vi "ReadVirtualSetup.vi"(8 "error in (no error)":errorcluster, 11 "Project.lvclass In":refnum<class "Project.lvclass">) -> (0 "error out":errorcluster, 2 "VirtualTypeData":T1={"Search Name"="", "Start X"=0.0, "Increase X"=0.0, "X Step"=1, "Start Y"=0.0, "Increase Y"=0.0, "Y Step"=1, "Sensor"=0} {"Y Step" min=1 step=1; "X Step" min=1 step=1}, 3 "Project.lvclass Out":refnum<class "Project.lvclass">)   [LabVIEW 2014, in "Project.lvclass"]
uses:
  Project.lvclass
  Virtual/Control/AllVirtualTypeData.ctl
  VirtualSetupDataTypeDefine.ctl
  Project.lvclass/Project.ctl
  Virtual/VirtualOrigin.lvclass
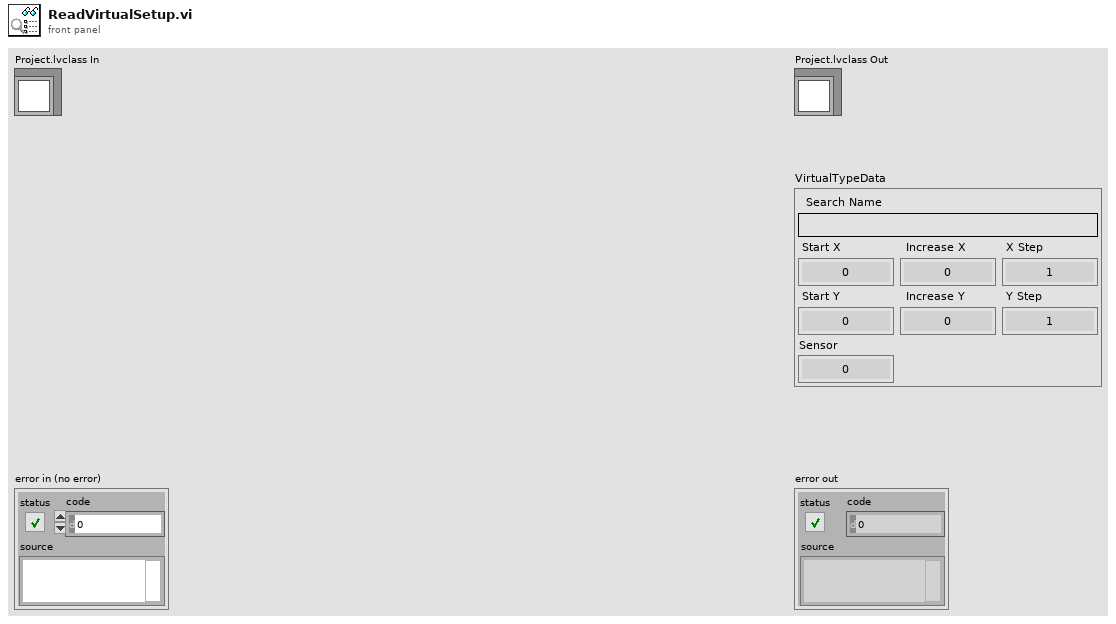
[diagram p1: front panel]
types:
  T1 = typedef "VirtualOrigin.lvclass/AllVirtualTypeData.ctl" = cluster{"Search Name":string, "Start X":dbl, "Increase X":dbl, "X Step":i32, "Start Y":dbl, "Increase Y":dbl, "Y Step":i32, "Sensor":i32}
  T2 = typedef "Project.lvclass/VirtualSetupDataTypeDefine.ctl" = T1[]
  T3 = typedef "Project.lvclass/ProjectDataTableTypeDefine.ctl" = string[][]
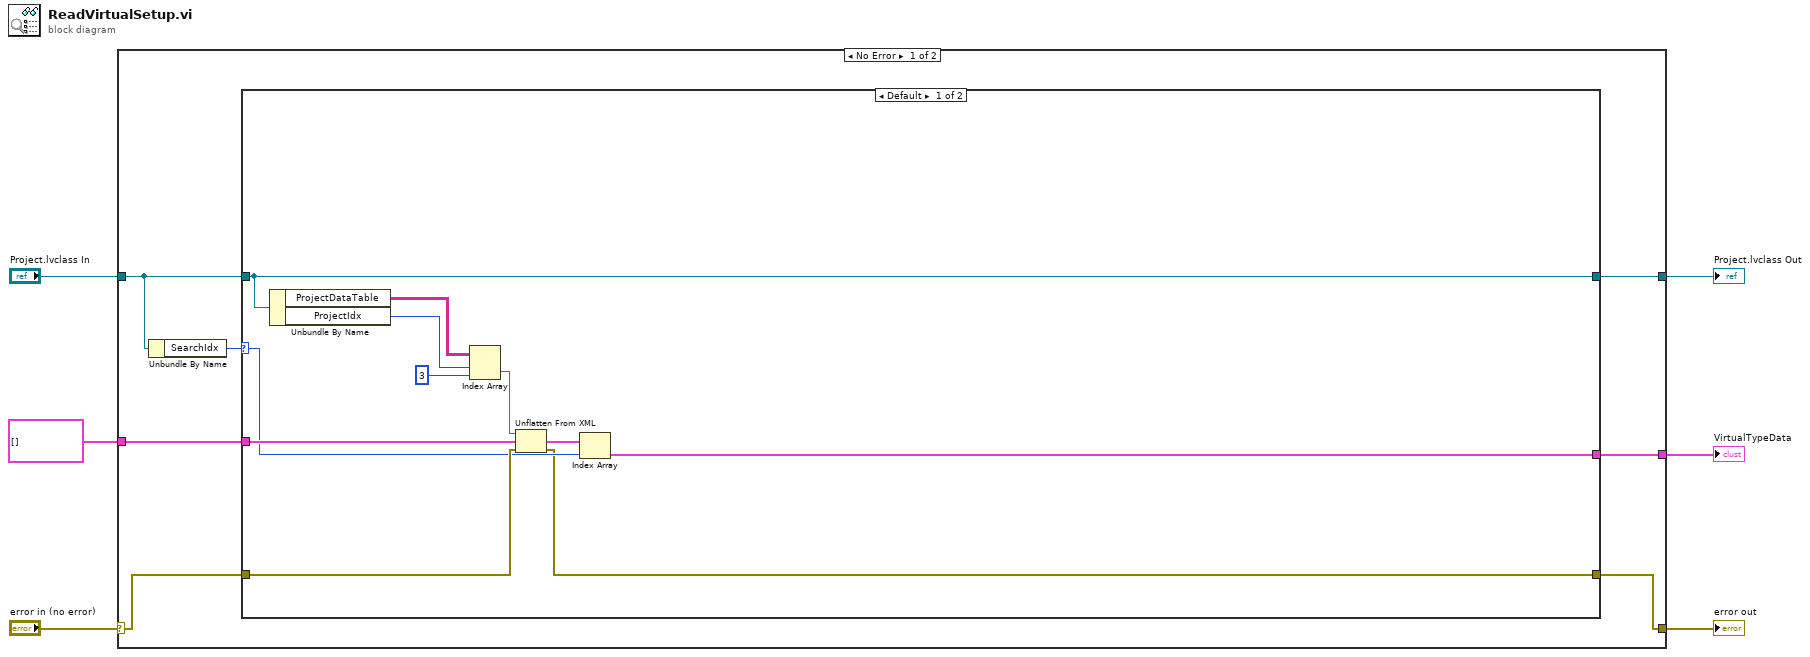
[diagram p0: block diagram]
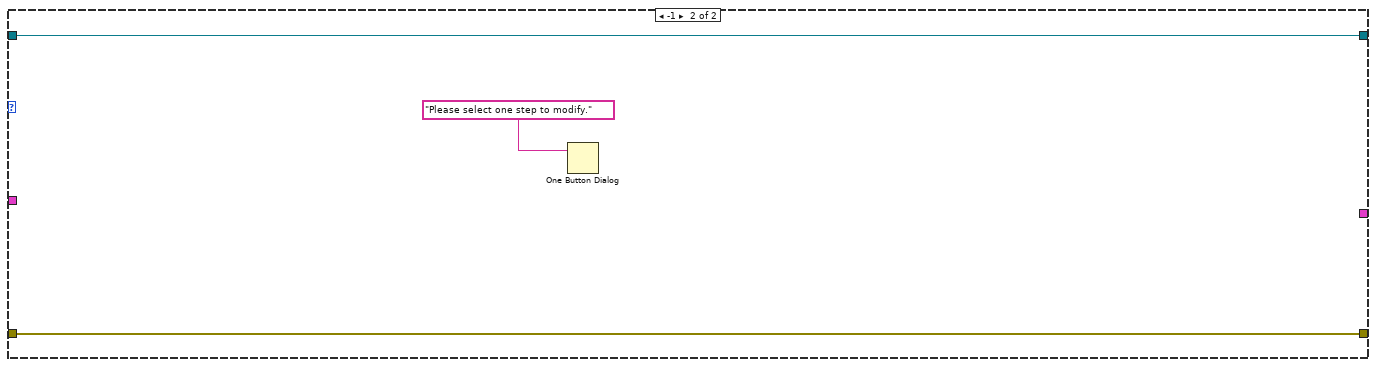
[diagram p2: hidden frame]
diagram:
  n1 = case shown="No Error" "error in (no error)" {
    selector: "error in (no error)" -> [w9 w29]
    tunnel: [w8 w29] -> w5
    tunnel: "Project.lvclass In" -> [w12 w28]
    tunnel: [w11 w28] -> w3
    tunnel: T2 [] ("VirtualSetupClusterArray") -> [w10 _]
    tunnel: [w7 _] -> w1
    frame No Error {
      n2 = Unbundle By Name(w12) -> ("SearchIdx"=w13:i32)
      n3 = case shown="Default" w13 {
        selector: w13 -> [w17 _]
        tunnel: w12 -> [w16 w27]
        tunnel: [w16 w27] -> w11
        tunnel: w10 -> [w23 _]
        tunnel: w9 -> [w18 w26]
        tunnel: [w15 w26] -> w8
        tunnel: [w14 _] -> w7
        frame Default {
          n4 = Unbundle By Name(w16) -> ("ProjectDataTable"=w22:T3, "ProjectIdx"=w21:i32)
          n5 = Index Array(array=w22, index (row)=w21, index (col)=3 ("disabled index (col)")) -> (element=w24:string)
          n6 = Unflatten From XML(xml string=w24, type=w23, error in (no error)=w18) -> (value=w19:T2, error out=w15:errorcluster)
          n7 = Index Array(array=w19, index=w17) -> (element=w14:T1)
        }
        frame -1 {
          n8 = One Button Dialog(message="Please select one step to modify.") -> ()  [unwired: 1 in, 1 out]
        }
      }
    }
    frame Error {
    }
  }
  "error out" <- w5
  "Project.lvclass Out" <- w3
  "VirtualTypeData" <- w1
